vi "analog_input.vi"() -> ()   [LabVIEW 2013]
uses:
  <vilib>/DAQmx/create/channels.llb/DAQmx Create Channel (AI-Voltage-Basic).vi
  <vilib>/DAQmx/configure/timing.llb/DAQmx Timing (Sample Clock).vi
  <vilib>/DAQmx/read.llb/DAQmx Read (Analog 1D Wfm NChan 1Samp).vi
  <vilib>/Utility/error.llb/DialogType.ctl
panel:
  in  "measurement delay":u32
  in  "error in":errorcluster
  in  "physical channels":tag="PXI1Slot7/ai0:2"
  out "Wattage chart":waveform(dbl)[](graph)=[{"t0"=timestamp(3432733595.521836 s since 1904-01-01), "dt"=0.01, "Y"=[9.068899858091251], "attributes"=variant("NI_ChannelName"=variant(string "PXI1Slot7/ai0"), "NI_UnitDescription"=variant(string "Volts"))}, {"t0"=timestamp(3432733595.521847 s since 1904-01-01), "dt"=0.01, "Y"=[5.945396887099972], "attributes"=variant("NI_ChannelName"=variant(string "PXI1Slot7/ai1"), "NI_UnitDescription"=variant(string "Volts"))}, {"t0"=timestamp(3432733595.5218577 s since 1904-01-01), "dt"=0.01, "Y"=[3.1289786148532777], "attributes"=variant("NI_ChannelName"=variant(string "PXI1Slot7/ai2"), "NI_UnitDescription"=variant(string "Volts"))}]
  in  "location":string[](array[string])=["out of SHG crystal", "before fiber", "after fiber"]
  out "voltage":dbl[](array[numeric])=[2.5261559493290395, 4.017160058851332, 0.6257957229706556]
  out "watts":dbl[](array[numeric])=[9.068899858091251, 5.945396887099972, 3.1289786148532777] format="%#_4g"
  in  "scaling":dbl[](array[numeric])=[3.59, 1.48, 5.0]
  in  "stop (F)":bool
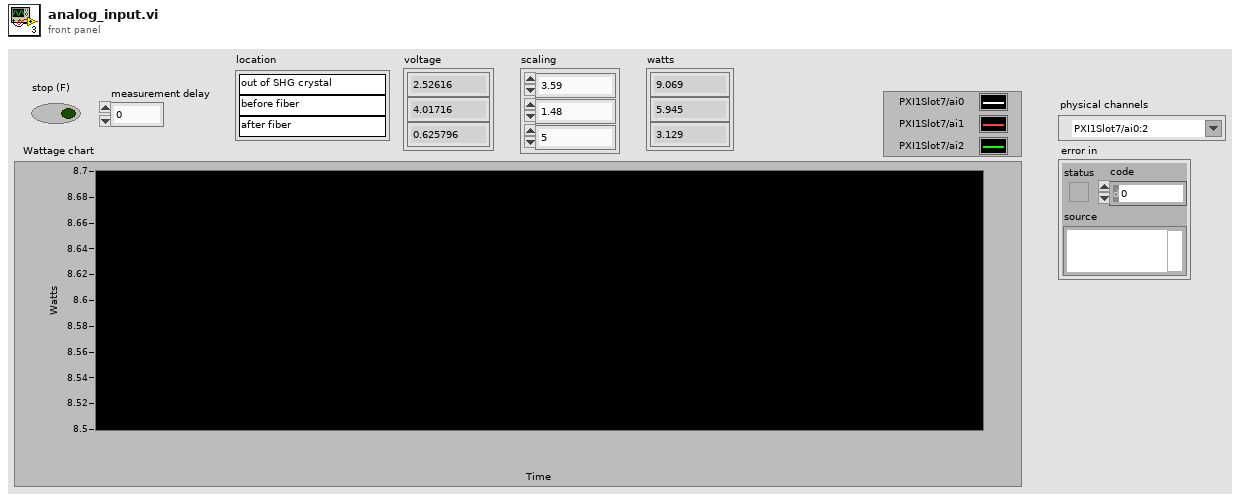
[diagram p1: front panel]
types:
  T1 = typedef "DialogType.ctl" = u16
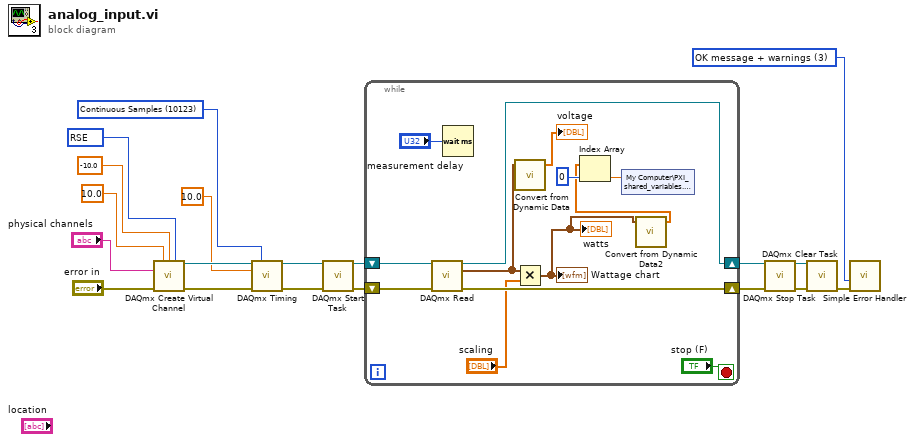
[diagram p0: block diagram]
diagram:
  w1 = T1 3 items=["no dialog", "OK message", "continue or stop message", "OK message + warnings", "continue/stop + warnings"] ("type of dialog (OK msg:1)")
  w7 = 10123 items=["Finite Samples"=10178, "Continuous Samples"=10123, "Hardware Timed Single Point"=12522] ("sample mode")
  w18 = 10083 items=["default"=-1, "RSE"=10083, "NRSE"=10078, "Differential"=10106, "Pseudodifferential"=12529] ("input terminal configuration")
  n1 = call-poly <vilib>:"DAQmx Create Virtual Channel.vi"("maximum value"=10.0, "minimum value"=-10.0, "input terminal configuration"=w18, "physical channels"="physical channels", "error in"="error in") -> ("task out"=w10:refnum<k21>, "error out"=w9:errorcluster)  [unwired: 9 in]
  n2 = call-poly <vilib>:"DAQmx Timing.vi"("task/channels in"=w10, "sample mode"=w7, "rate"=10.0, "error in"=w9) -> ("task out"=w3:refnum<k21>, "error out"=w4:errorcluster)  [unwired: 10 in]
  n3 = call <vilib>:"DAQmx Start Task.vi"("task/channels in"=w3, "error in"=w4) -> ("task out"=w12:refnum<k21>, "error out"=w14:errorcluster)  [unwired: 12 in]
  n4 = while {
    shift-right: [w27] -> w13
    shift-left: w14 -> [w29]
    shift-right: [w26] -> w11
    shift-left: w12 -> [w30]
    stop <- "stop (F)" stop-if-true
    n5 = call-poly <vilib>:"DAQmx Read.vi"("task/channels in"=w30, "error in"=w29) -> ("task out"=w26:refnum<k21>, "data"=w23:waveform(dbl)[], "error out"=w27:errorcluster)  [unwired: 11 in]
    n6 = Wait (ms)(milliseconds to wait="measurement delay") -> ()  [unwired: 1 out]
    n7 = call "Convert from Dynamic Data"("Dynamic Data Type"=w23) -> ("Array"=→"voltage":dbl[])  [unwired: 3 in]
    n8 = Multiply(x=w23, y="scaling") -> (x*y=w21:waveform(dbl)[])
    "watts" <- w21
    "Wattage chart" <- w21
    n9 = call "Convert from Dynamic Data2"("Dynamic Data Type"=w21) -> ("Array"=w20:dbl[])  [unwired: 3 in]
    n10 = Index Array(array=w20, index=0) -> (element=w31:dbl)
    n11 = shared-variable "My Computer\\PXI_shared_variables.lvlib\\watts"(w31) -> ()  [unwired: 1 in, 1 out]
  }
  n12 = call <vilib>:"DAQmx Stop Task.vi"("task/channels in"=w11, "error in"=w13) -> ("task out"=w15:refnum<k21>, "error out"=w16:errorcluster)  [unwired: 12 in]
  n13 = call <vilib>:"DAQmx Clear Task.vi"("task in"=w15, "error in"=w16) -> ("error out"=w2:errorcluster)  [unwired: 13 in]
  n14 = call <vilib>:"Simple Error Handler.vi"("type of dialog (OK msg:1)"=w1, "error in (no error)"=w2) -> ()  [unwired: 3 in, 5 out]
